vi "DSF.Shared.Configuration.Transfer.Channel Array to Blocks.vi"(8 "error in (no error)":errorcluster, 10 "Channel Descriptors":T2[](array[typedef]) {"base address" format="%016x"; "Channel Parameters"."offset" format="%d bytes"}, 11 "Transfer Configuration in":refnum<class "DSF.Shared.Configuration.Transfer.lvclass">) -> (0 "error out":errorcluster, 2 "Channel Block Descriptors":T1[](array[typedef]) {"count" format="%d elements"; "First Channel Descriptor"."base address" format="%016x"; "First Channel Descriptor"."Channel Parameters"."offset" format="%d bytes"}, 3 "Transfer Configuration out":refnum<class "DSF.Shared.Configuration.Transfer.lvclass">)   [LabVIEW 2017, in "DSF.Shared.lvlib" / "DSF.Shared.Configuration.Transfer.lvclass"]
uses:
  DSF.Shared.Configuration.Transfer.lvclass
  Typedefs/DSF.Shared.Typedefs.Configuration.Transfer.Channel Descriptor.ctl
  Typedefs/DSF.Shared.Typedefs.Configuration.Transfer.Channel Parameters.ctl
  Typedefs/DSF.Shared.Typedefs.Data Type.ctl
  Typedefs/DSF.Shared.Typedefs.Configuration.Transfer.Channel Block Descriptor.ctl
  DSF.Shared.lvlib
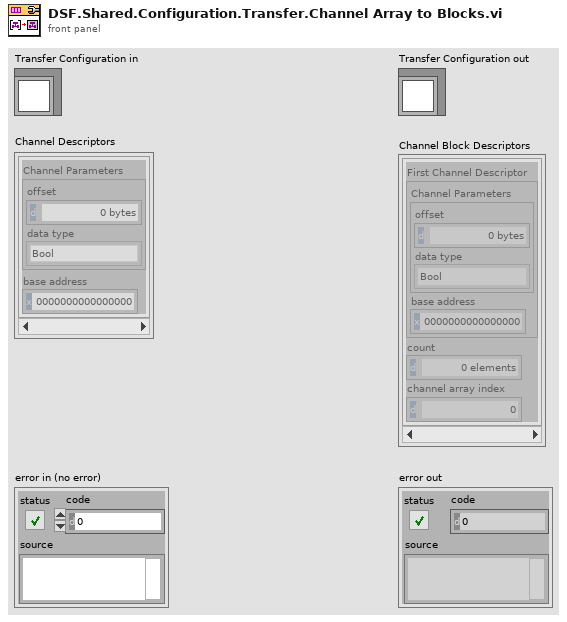
[diagram p1: front panel]
types:
  T1 = typedef "DSF.Shared.lvlib/DSF.Shared.Typedefs.Configuration.Transfer.Channel Block Descriptor.ctl" = cluster{"First Channel Descriptor":T2, "count":u64, "channel array index":u64}
  T2 = typedef "DSF.Shared.lvlib/DSF.Shared.Typedefs.Configuration.Transfer.Channel Descriptor.ctl" = cluster{"Channel Parameters":T3, "base address":u64}
  T3 = typedef "DSF.Shared.lvlib/DSF.Shared.Typedefs.Configuration.Transfer.Channel Parameters.ctl" = cluster{"offset":u64, "data type":T4}
  T4 = typedef "DSF.Shared.lvlib/DSF.Shared.Typedefs.Data Type.ctl" = enum8{"Bool", "SGL", "DBL", "I8", "I16", "I32", "I64", "U8", "U16", "U32", "U64"}
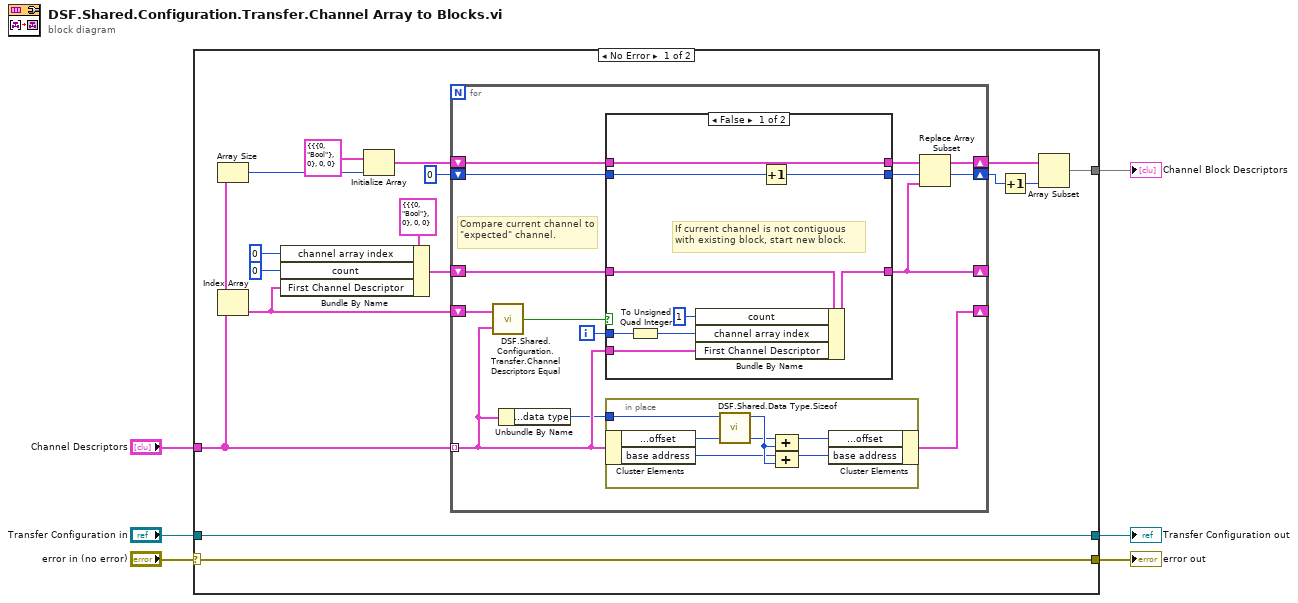
[diagram p0: block diagram]
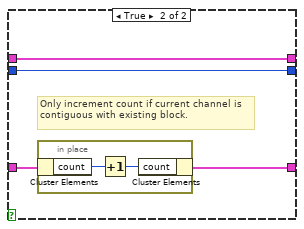
[diagram p2: hidden frame]
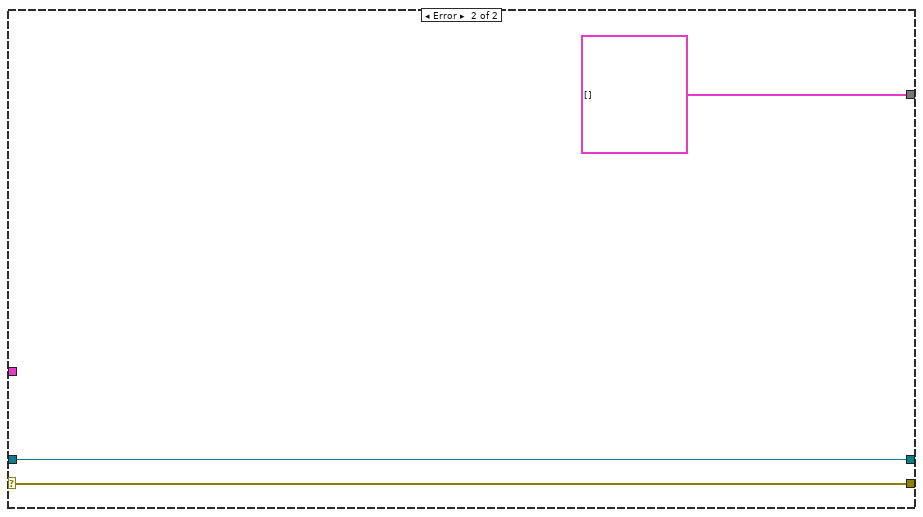
[diagram p3: hidden frame]
diagram:
  n1 = case shown="No Error" "error in (no error)" {
    selector: "error in (no error)" -> [w9 w59]
    tunnel: [w16 T1[] []] -> w6
    tunnel: "Channel Descriptors" -> [w7 _]
    tunnel: [w9 w59] -> w5
    tunnel: "Transfer Configuration in" -> [w8 w58]
    tunnel: [w8 w58] -> w4
    frame No Error {
      n2 = Array Size(array=w7) -> (size(s)=w21:i32)
      n3 = Index Array(array=w7) -> (element=w14:T2)  [unwired: 1 in]
      n4 = Bundle By Name(cluster=T1 {"First Channel Descriptor"={"Channel Parameters"={"offset"=0, "data type"=enum."Bool"}, "base address"=0}, "count"=0, "channel array index"=0} ("Channel Parameters"), "channel array index"=u64 0 ("index"), "count"=u64 0, "First Channel Descriptor"=w14) -> (w13:T1)
      n5 = Initialize Array(T1 {"First Channel Descriptor"={"Channel Parameters"={"offset"=0, "data type"=enum."Bool"}, "base address"=0}, "count"=0, "channel array index"=0} ("Channel Parameters"), w21) -> (w20:T1[])
      n6 = for {
        tunnel: w7 -> [w25] mode=indexing
        shift-right: [w27] -> _
        shift-left: w14 -> [w26]
        shift-right: [w32] -> w18
        shift-left: w20 -> [w35]
        shift-right: [w31] -> w17
        shift-left: 0 ("size(s)") -> [w34]
        shift-right: [w30] -> _
        shift-left: w13 -> [w29]
        i -> [w28]
        # "Compare current channel to \"expected\" channel."
        n7 = call "DSF.Shared.Configuration.Transfer.Channel Descriptors Equal.vi"("Channel Descriptor 2"=w25, "Channel Descriptor 1"=w26) -> ("equal?"=w24:bool)
        n8 = Unbundle By Name(w25) -> ("Channel Parameters.data type"=w23:T4)
        n9 = case shown="False" w24 {
          tunnel: w29 -> [w48 w54]
          tunnel: [w42 w53] -> w30
          tunnel: w35 -> [w49 w52]
          tunnel: w34 -> [w50 w51]
          tunnel: [w47 w51] -> w31
          tunnel: [w49 w52] -> w33
          tunnel: w25 -> [w46 _]
          tunnel: w28 -> [w45 _]
          frame False {
            # "If current channel is not contiguous with existing block, start new block."
            n10 = To Unsigned Quad Integer(1:w45) -> (0:w43:u64)
            n11 = Bundle By Name(cluster=w48, "count"=u64 1, "channel array index"=w43, "First Channel Descriptor"=w46) -> (w42:T1)
            n12 = Increment(x=w50) -> (x+1=w47:i32)
          }
          frame True {
            # "Only increment count if current channel is contiguous with existing block."
            n13 = in-place {
              n14 = in-place-cluster #1(w54) -> ("count"=w56:u64)
              n15 = Increment(x=w56) -> (x+1=w55:u64)
              n16 = in-place-cluster #1("count"=w55) -> (w53:T1)
            }
          }
        }
        n17 = in-place {
          in-place-border: w23 -> [w37]
          n18 = in-place-cluster #2(w25) -> ("Channel Parameters.offset"=w39:u64, "base address"=w40:u64)
          n19 = call "DSF.Shared.Data Type.Sizeof.vi"("data type"=w37) -> ("size in bytes"=w41:u64)  [unwired: 9 in, 1 out]
          n20 = Compound Arithmetic op=ADD(w39, w41) -> (w36:u64)
          n21 = Compound Arithmetic op=ADD(w40, w41) -> (w38:u64)
          n22 = in-place-cluster #2("Channel Parameters.offset"=w36, "base address"=w38) -> (w27:T2)
        }
        n23 = Replace Array Subset(array=w33, new element=w30, index=w31) -> (w32:T1[])
      }
      n24 = Increment(x=w17) -> (x+1=w11:i32)
      n25 = Array Subset(array=w18, length=w11) -> (w16:T1[])  [unwired: 1 in]
    }
    frame Error {
    }
  }
  "Channel Block Descriptors" <- w6
  "error out" <- w5
  "Transfer Configuration out" <- w4
